vi "Begin.vi"(8 "error in":errorcluster) -> (0 "error out":errorcluster)   [LabVIEW 2017]
doc: "Called before other user functions, this VI is expected to open initial I/O refnums, load in file data, and do all program initialization. Notice that the <B>error out</B> terminal is simply used for data flow. Wiring it to other structures or subVIs ensures that this VI runs first."
uses:
  <vilib>/Rock Robotics/WPI/DriverStation/WPI_DriverStationRobotMode2.ctl
  <vilib>/Rock Robotics/SystemInterfaces/DIO/FPGA_DIOPWMChannel.ctl
  <vilib>/Rock Robotics/WPI/Joystick/WPI_JoystickDeviceEnum.ctl
  <vilib>/Rock Robotics/SystemInterfaces/DIO/FPGA_DIOChannel.ctl
  <vilib>/Rock Robotics/SystemInterfaces/AI/FPGA_AIChannel.ctl
  <vilib>/Rock Robotics/WPI/Solenoid/WPI_SolenoidChannel.ctl
  Robot Global Data.vi
  <vilib>/Rock Robotics/WPI/MotorControl/WPI_MotorControlOpen Talon.vi
  <vilib>/Rock Robotics/WPI/Switch/WPI_SwitchOpenLimit.vi
  <vilib>/Rock Robotics/WPI/Solenoid/WPI_SolenoidOpenDouble.vi
  <vilib>/Rock Robotics/WPI/MotorControl/WPI_MotorControlOpen VictorSP.vi
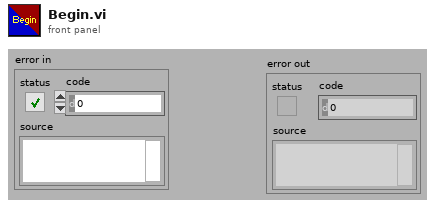
[diagram p1: front panel]
types:
  T1 = typedef "FPGA_DIOPWMChannel.ctl" = enum8{"PWM 0", "PWM 1", "PWM 2", "PWM 3", "PWM 4", "PWM 5", "PWM 6", "PWM 7", "PWM 8", "PWM 9", "PWM MXP 0", "PWM MXP 1", "PWM MXP 2", "PWM MXP 3", "PWM MXP 4", "PWM MXP 5", "PWM MXP 6", "PWM MXP 7", "PWM MXP 8", "PWM MXP 9", "Invalid"}
  T2 = typedef "WPI_SolenoidChannel.ctl" = enum8{"Solenoid 0", "Solenoid 1", "Solenoid 2", "Solenoid 3", "Solenoid 4", "Solenoid 5", "Solenoid 6", "Solenoid 7", "Invalid"}
  T3 = typedef "FPGA_DIOChannel.ctl" = enum8{"DIO 0", "DIO 1", "DIO 2", "DIO 3", "DIO 4", "DIO 5", "DIO 6", "DIO 7", "DIO 8", "DIO 9", "DIO MXP 0", "DIO MXP 1", "DIO MXP 2", "DIO MXP 3", "DIO MXP 4", "DIO MXP 5", "DIO MXP 6", "DIO MXP 7", "DIO MXP 8", "DIO MXP 9", "DIO MXP 10", "DIO MXP 11", "DIO MXP 12", "DIO MXP 13", "DIO MXP 14", "DIO MXP 15", "SPI Port CS1", "SPI Port CS2", "SPI Port CS3", "SPI Port MISO", "SPI Port MOSI", "Invalid"}
  T4 = typedef "WPI_JoystickDeviceEnum.ctl" = enum16{"USB 0", "USB 1", "USB 2", "USB 3", "USB 4", "USB 5"}
  T5 = typedef "FPGA_AIChannel.ctl" = enum8{"AI 0", "AI 1", "AI 2", "AI 3", "AI MXP 0", "AI MXP 1", "AI MXP 2", "AI MXP 3", "Invalid"}
  T6 = typedef "WPI_DriverStationRobotMode2.ctl" = enum16{"Autonomous Disabled", "Autonomous Enabled", "Teleop Disabled", "Teleop Enabled", "Disconnected", "Finish", "Test Disabled", "Test Enabled", "Emergency Stopped"}
  T7 = typedef "WPI_MotorControlDeviceRef.ctl" = cluster{"DeviceStatus":errorcluster, "Type":T8, "PWM":cluster{"PWM Channel":T1, "DeadBand":T9}, "CAN":cluster{"Device Number":u8, "SetOutput VI Ref":variant, "GetOutput VI Ref":variant, "Enable VI Ref":variant, "Disable VI Ref":variant, "Data":variant}, "Invert":bool, "DIO PWM":cluster{"PWM \"Enable\" Channel":T1, "DIOChannel":T3, "PWM Rate":dbl}}
  T8 = typedef "WPI_MotorControlType.ctl" = enum16{"PWM", "CAN", "DIO PWM"}
  T9 = typedef "WPI_PWMDeadband.ctl" = cluster{"Name":string, "maxPositivePwm":i32, "minPositivePwm":i32, "centerPwm":i32, "maxNegativePwm":i32, "minNegativePwm":i32, "angularRange":u16}
  T10 = typedef "WPI_SolenoidDevRef.ctl" = cluster{"DevStatus":errorcluster, "Pneumatics Control Module":u8, "Forward Solenoid Channel":T2, "Reverse Solenoid Channel":T2}
  T11 = typedef "WPI_AnalogChannelDevRef.ctl" = cluster{"DevStatus":errorcluster, "Analog Channel":T5}
  T12 = typedef "WPI_SwitchDevRef.ctl" = cluster{"DevStatus":errorcluster, "DIO Channel":T3, "CntIndex":T13, "Normally Closed":bool}
  T13 = typedef "FPGA_CounterCtrSystemIndex.ctl" = enum8{"Ctr 0", "Ctr 1", "Ctr 2", "Ctr 3", "Ctr 4", "Ctr 5", "Ctr 6", "Ctr 7", "Invalid"}
  T14 = typedef "WPI_JoystickDevRef.ctl" = cluster{"Device":T4}
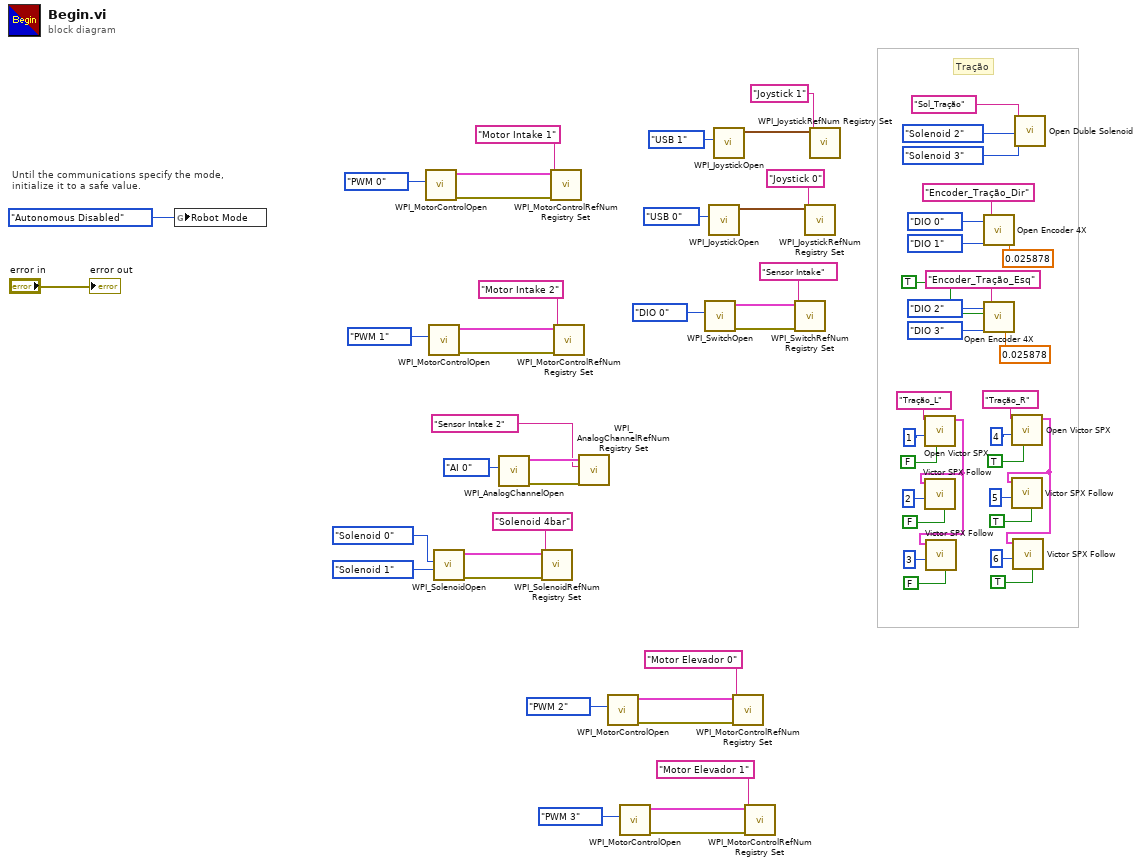
[diagram p0: block diagram]
diagram:
  # "Tração"
  # "Until the communications specify the mode,\ninitialize it to a safe value."
  n1 = global write "Robot Global Data.vi" "Robot Mode"(WPI_DriverStationRobotMode2."Autonomous Disabled" ("Robot Mode")) -> ()
  n2 = call-poly <vilib>:"WPI_MotorControlOpen.vi"("PWM Channel"=FPGA_DIOPWMChannel."PWM 0") -> ("error out"=w62:errorcluster, "MotorControlDeviceRef"=w63:T7)  [unwired: 9 in]
  n3 = call-poly <vilib>:"WPI_MotorControlOpen.vi"("PWM Channel"=FPGA_DIOPWMChannel."PWM 1") -> ("error out"=w58:errorcluster, "MotorControlDeviceRef"=w59:T7)  [unwired: 9 in]
  n4 = call-poly <vilib>:"WPI_SolenoidOpen.vi"("Reverse Solenoid Channel"=WPI_SolenoidChannel."Solenoid 1", "Forward Solenoid Channel"=WPI_SolenoidChannel."Solenoid 0") -> ("error out"=w12:errorcluster, "SolenoidDevRef"=w13:T10)  [unwired: 8 in]
  n5 = call <vilib>:"WPI_AnalogChannelOpen.vi"("Analog Channel"=FPGA_AIChannel."AI 0") -> ("error out"=w47:errorcluster, "AIDeviceRef"=w48:T11)  [unwired: 9 in]
  n6 = call <vilib>:"WPI_SolenoidRefNum Registry Set.vi"("error in (no error)"=w12, "refnum name"="Solenoid 4bar", "SolenoidDevRef"=w13) -> ()  [unwired: 7 in, 2 out]
  n7 = call <vilib>:"WPI_MotorControlRefNum Registry Set.vi"("error in (no error)"=w62, "refnum name"="Motor Intake 1", "MotorControlDevRef"=w63) -> ()  [unwired: 7 in, 2 out]
  n8 = call <vilib>:"WPI_MotorControlRefNum Registry Set.vi"("error in (no error)"=w58, "refnum name"="Motor Intake 2", "MotorControlDevRef"=w59) -> ()  [unwired: 7 in, 2 out]
  n9 = call <vilib>:"WPI_AnalogChannelRefNum Registry Set.vi"("error in (no error)"=w47, "refnum name"="Sensor Intake 2", "AIDeviceRef"=w48) -> ()  [unwired: 7 in, 2 out]
  n10 = call-poly <vilib>:"WPI_MotorControlOpen.vi"("PWM Channel"=FPGA_DIOPWMChannel."PWM 2") -> ("error out"=w7:errorcluster, "MotorControlDeviceRef"=w8:T7)  [unwired: 9 in]
  n11 = call-poly <vilib>:"WPI_MotorControlOpen.vi"("PWM Channel"=FPGA_DIOPWMChannel."PWM 3") -> ("error out"=w2:errorcluster, "MotorControlDeviceRef"=w1:T7)  [unwired: 9 in]
  n12 = call-poly <vilib>:"WPI_SwitchOpen.vi"("DIO Channel"=FPGA_DIOChannel."DIO 0") -> ("error out"=w50:errorcluster, "SwitchDevRef"=w51:T12)  [unwired: 9 in]
  n13 = call <vilib>:"WPI_JoystickOpen.vi"("JoystickDevice"=WPI_JoystickDeviceEnum."USB 0") -> ("JoystickDevRef"=w42:T14)  [unwired: 10 in]
  n14 = call <vilib>:"WPI_JoystickOpen.vi"("JoystickDevice"=WPI_JoystickDeviceEnum."USB 1") -> ("JoystickDevRef"=w55:T14)  [unwired: 10 in]
  n15 = call <vilib>:"WPI_MotorControlRefNum Registry Set.vi"("error in (no error)"=w7, "refnum name"="Motor Elevador 0", "MotorControlDevRef"=w8) -> ()  [unwired: 7 in, 2 out]
  n16 = call <vilib>:"WPI_MotorControlRefNum Registry Set.vi"("error in (no error)"=w2, "refnum name"="Motor Elevador 1", "MotorControlDevRef"=w1) -> ()  [unwired: 7 in, 2 out]
  n17 = call <vilib>:"WPI_SwitchRefNum Registry Set.vi"("error in (no error)"=w50, "refnum name"="Sensor Intake", "SwitchDevRef"=w51) -> ()  [unwired: 7 in, 2 out]
  n18 = call <vilib>:"WPI_JoystickRefNum Registry Set.vi"("refnum name"="Joystick 0", "JoystickDevRef"=w42) -> ()  [unwired: 8 in, 2 out]
  n19 = call <vilib>:"WPI_JoystickRefNum Registry Set.vi"("refnum name"="Joystick 1", "JoystickDevRef"=w55) -> ()  [unwired: 8 in, 2 out]
  n20 = call "Open Victor SPX.vi"("Invert"=FALSE, "Device Number"=u8 1, "refnum name"="Tração_L") -> ("PhoenixMotorControlDevRef"=w27:T7)  [unwired: 8 in]
  n21 = call "Victor SPX Follow.vi"("Master Controller to Follow"=w27, "Device Number"=u8 2, "Invert"=FALSE) -> ()  [unwired: 7 in]
  n22 = call "Victor SPX Follow.vi"("Master Controller to Follow"=w27, "Device Number"=u8 3, "Invert"=FALSE) -> ()  [unwired: 7 in]
  n23 = call "Open Encoder 4X.vi"("DistancePerCount"=0.025878, "B Channel"=FPGA_DIOChannel."DIO 0", "A Channel"=FPGA_DIOChannel."DIO 1", "refnum name"="Encoder_Tração_Dir") -> ()  [unwired: 2 in]
  n24 = call "Open Encoder 4X.vi"("DistancePerCount"=0.025878, "B Channel"=FPGA_DIOChannel."DIO 2", "A Channel"=FPGA_DIOChannel."DIO 3", "Invert Direction (False)"=TRUE, "refnum name"="Encoder_Tração_Esq") -> ()  [unwired: 1 in]
  n25 = call "Open Victor SPX.vi"("Invert"=TRUE, "Device Number"=u8 4, "refnum name"="Tração_R") -> ("PhoenixMotorControlDevRef"=w19:T7)  [unwired: 8 in]
  n26 = call "Victor SPX Follow.vi"("Master Controller to Follow"=w19, "Device Number"=u8 5, "Invert"=TRUE) -> ()  [unwired: 7 in]
  n27 = call "Victor SPX Follow.vi"("Master Controller to Follow"=w19, "Device Number"=u8 6, "Invert"=TRUE) -> ()  [unwired: 7 in]
  n28 = call "Open Duble Solenoid.vi"("Reverse Solenoid Channel"=WPI_SolenoidChannel."Solenoid 3", "Forward Solenoid Channel"=WPI_SolenoidChannel."Solenoid 2", "refnum name"="Sol_Tração") -> ()  [unwired: 9 in]
  "error out" <- "error in"
